vi "Test.vi"() -> ()   [LabVIEW 2013]
uses:
  <vilib>/FieldPoint/FP Close.llb/FP Close.vi
  <vilib>/FieldPoint/Polymorphic Write.llb/FP Write (Boolean).vi
  <vilib>/FieldPoint/Polymorphic Read.llb/FP Read (Boolean).vi
panel:
  in  "value 2":bool=TRUE
  out "value":bool
  out "error out":errorcluster
  in  "stop":bool
  in  "item name":string="Channel 0"
  in  "device name":string="cFP-AI-112 @1"
  in  "comm resource name":string="NDCXIIBRK2RIO3"
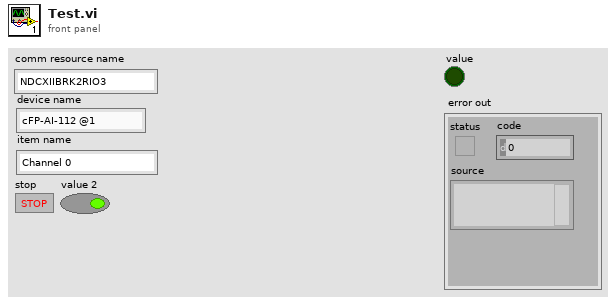
[diagram p1: front panel]
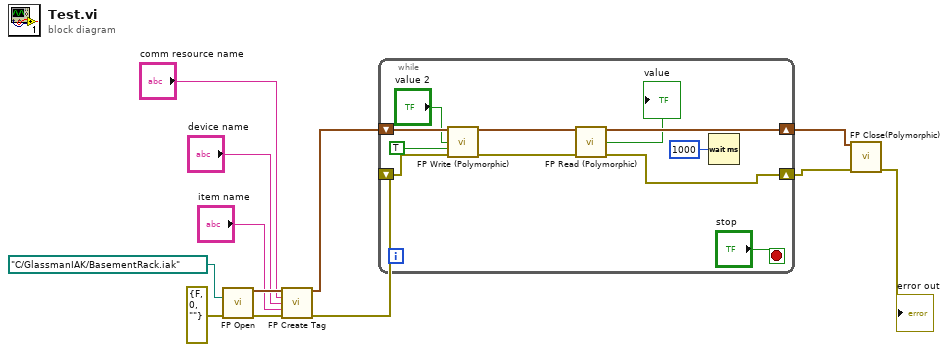
[diagram p0: block diagram]
diagram:
  n1 = call <vilib>:"FP Open.vi"("iak file path"=path "C:/GlassmanIAK/BasementRack.iak", "error in (no error)"=errorcluster {"status"=FALSE, "code"=0, "source"=""}) -> ("FP refnum out"=w11:cluster{"server refnum":u32, "tag refnum":u32}, "error out"=w7:errorcluster)  [unwired: 12 in]
  n2 = call <vilib>:"FP Create Tag.vi"("FP refnum in"=w11, "comm resource name"="comm resource name", "device name"="device name", "item name"="item name", "error in (no error)"=w7) -> ("FP refnum out"=w5:cluster{"server refnum":u32, "tag refnum":u32}, "error out"=w4:errorcluster)  [unwired: 9 in]
  n3 = while {
    shift-right: [w20] -> w3
    shift-left: w4 -> [w16]
    shift-right: [w21] -> w2
    shift-left: w5 -> [w19]
    stop <- "stop" stop-if-true
    n4 = call-poly <vilib>:"FP Write (Polymorphic).vi"("FP refnum in"=w19, "value"="value 2", "on change (false)"=TRUE, "error in (no error)"=w16) -> ("FP refnum out"=w18:cluster{"server refnum":u32, "tag refnum":u32}, "error out"=w17:errorcluster)  [unwired: 9 in, 1 out]
    n5 = call-poly <vilib>:"FP Read (Polymorphic).vi"("FP refnum in"=w18, "error in (no error)"=w17) -> ("FP refnum out"=w21:cluster{"server refnum":u32, "tag refnum":u32}, "value"=→"value":bool, "error out"=w20:errorcluster)  [unwired: 10 in, 1 out]
    n6 = Wait (ms)(milliseconds to wait=u32 1000) -> ()  [unwired: 1 out]
  }
  n7 = call-poly <vilib>:"FP Close(Polymorphic).vi"("FP refnum in"=w2, "error in (no error)"=w3) -> ("error out"=→"error out":errorcluster)  [unwired: 13 in]
